vi "Draw.vi"(8 "error in (no error)":errorcluster, 10 "2D Picture in":picture, 11 "TriangleB in":refnum<class "TriangleB.lvclass">) -> (0 "error out":errorcluster, 2 "2D Picture out":picture, 3 "TriangleB out":refnum<class "TriangleB.lvclass">)   [LabVIEW 2021, in "Picture2D.lvlib" / "TriangleB.lvclass"]
uses:
  TriangleB.lvclass
  C:/Users/Dany/OneDrive/LabVIEW/Class/Picture2D/Shape/Shape.lvclass
  C:/Users/Dany/OneDrive/LabVIEW/Class/Picture2D/Triangle/Triangle.lvclass
  C:/Users/Dany/OneDrive/LabVIEW/Class/Picture2D/Polygone/Polygone.lvclass
  Pen/Pen.lvclass
  Color/Color.lvclass
  Point/Point.lvclass
  TriangleB.lvclass/TriangleB.ctl
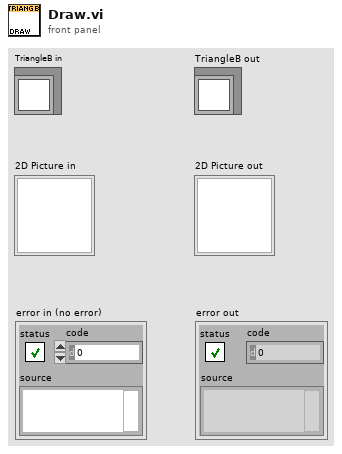
[diagram p1: front panel]
types:
  T1 = cluster{"Width":u16, "Style":enum32{"Solid", "Dash", "Dot", "DashDot", "DashDotDot"}}
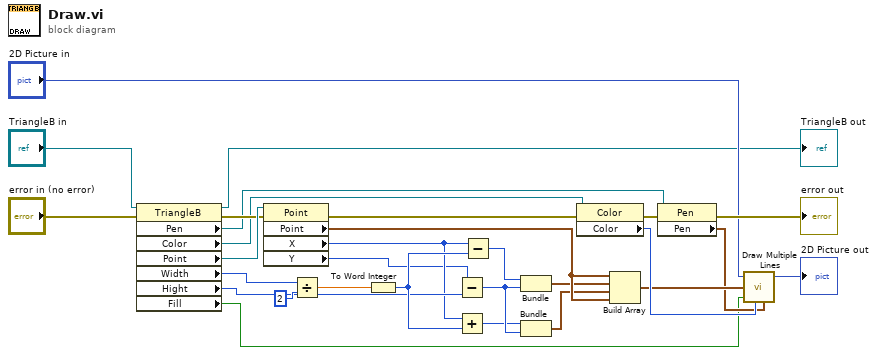
[diagram p0: block diagram]
diagram:
  n1 = property class="TriangleB"(reference="TriangleB in", error in="error in (no error)") -> (reference out=→"TriangleB out":refnum<class "TriangleB.lvclass">, error out=w28:errorcluster, "Pen"=w25:refnum<class "Pen.lvclass">, "Color"=w24:refnum<class "Color.lvclass">, "Point"=w29:refnum<class "Point.lvclass">, "Width"=w15:i16, "Hight"=w5:i16, "Fill"=w19:bool)
  n2 = property class="Point"(reference=w29, error in=w28) -> (error out=w27:errorcluster, "Point"=w22:cluster{"x":i16, "y":i16}, "X"=w2:i16, "Y"=w1:i16)  [unwired: 1 out]
  n3 = Divide(x=w15, y=i16 2) -> (x/y=w13:dbl)
  n4 = To Word Integer(number=w13) -> (16bit integer=w7:i16)
  n5 = Subtract(x=w1, y=w5) -> (x-y=w4:i16)
  n6 = Add(x=w2, y=w7) -> (x+y=w3:i16)
  n7 = Subtract(x=w2, y=w7) -> (x-y=w6:i16)
  n8 = Bundle(w6, w4) -> (w16:cluster{i16, i16})  [unwired: 1 in]
  n9 = Bundle(w3, w4) -> (w12:cluster{i16, i16})  [unwired: 1 in]
  n10 = property class="Color"(reference=w24, error in=w27) -> (error out=w26:errorcluster, "Color"=w23:u32)  [unwired: 1 out]
  n11 = Build Array(w22, w16, w12, w22) -> (w21:cluster{"x":i16, "y":i16}[])
  n12 = property class="Pen"(reference=w25, error in=w26) -> (error out=→"error out":errorcluster, "Pen"=w20:T1)  [unwired: 1 out]
  n13 = call <vilib>:"Draw Multiple Lines.vi"("picture"="2D Picture in", "line endpoints"=w21, "fill?(F)"=w19, "color(black)"=w23, "pen"=w20) -> ("new picture"=→"2D Picture out":picture)  [unwired: 4 in]
